vi "ActualizarTabla.vi"(8 "error in (no error)":errorcluster, 11 "Soda Actor in":refnum<class "Soda Actor.lvclass">) -> (0 "error out":errorcluster, 3 "Soda Actor out":refnum<class "Soda Actor.lvclass">)   [LabVIEW 2019, in "Soda Actor.lvlib" / "Soda Actor.lvclass"]
uses:
  Soda Actor.lvclass
  Soda Actor.lvclass/Soda Actor.ctl
  <vilib>/Utility/config.llb/Read Key (Double).vi
  <vilib>/Utility/config.llb/Read Key (String).vi
  <vilib>/Utility/config.llb/NI_LVConfig.lvlib
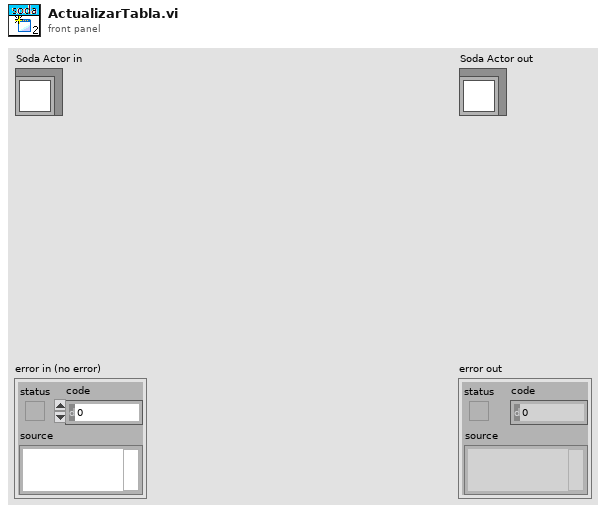
[diagram p1: front panel]
types:
  T1 = typedef "NI_LVConfig.lvlib/Config Data RefNum.ctl" = refnum<k1>
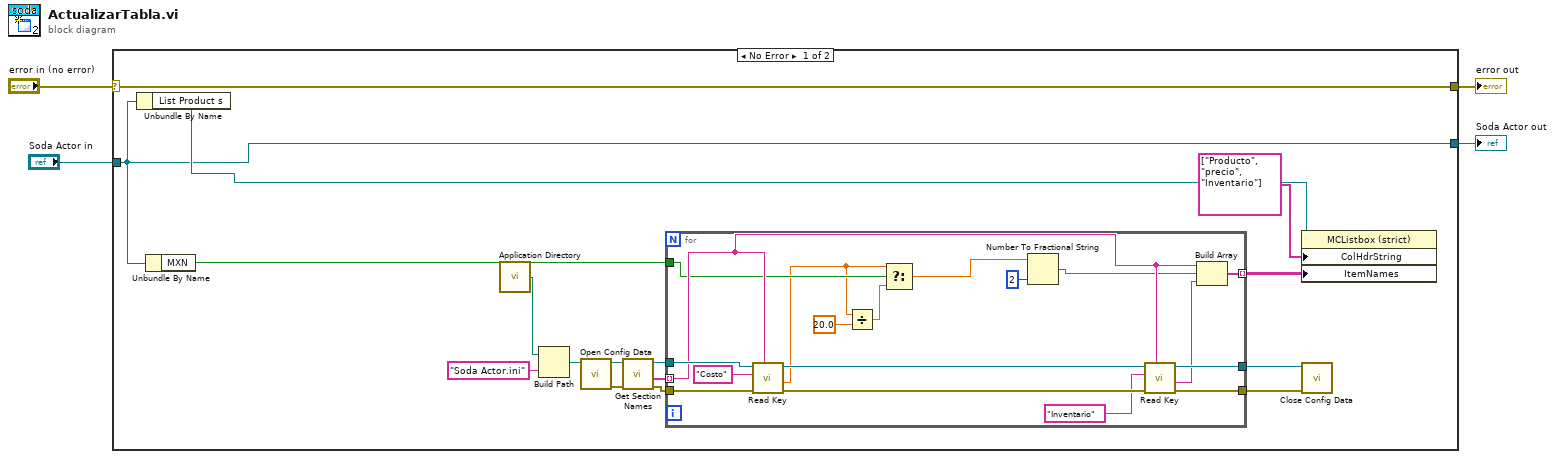
[diagram p0: block diagram]
diagram:
  n1 = case shown="No Error" "error in (no error)" {
    selector: "error in (no error)" -> [w6 w40]
    tunnel: [w6 w40] -> w3
    tunnel: [w15 w39] -> w1
    tunnel: "Soda Actor in" -> [w15 w39]
    frame No Error {
      n2 = Unbundle By Name(w15) -> ("List Product s"=w20:refnum<vi>)
      n3 = Unbundle By Name(w15) -> ("MXN"=w14:bool)
      n4 = call <vilib>:"Application Directory.vi"() -> ("Application Directory"=w19:path)
      n5 = Build Path(base path=w19, name or relative path="Soda Actor.ini") -> (appended path=w18:path)
      n6 = call <vilib>:"Open Config Data.vi"("configuration file path"=w18) -> ("error out"=w11:errorcluster, "refnum"=w12:T1)  [unwired: 8 in, 1 out]
      n7 = call <vilib>:"Get Section Names.vi"("error in (no error)"=w11, "refnum"=w12) -> ("error out"=w9:errorcluster, "section names"=w8:string[], "refnum out"=w10:T1)  [unwired: 7 in]
      n8 = for {
        tunnel: w9 -> [w37]
        tunnel: w10 -> [w38]
        tunnel: [w34] -> w16
        tunnel: [w33] -> w17
        tunnel: w14 -> [w24]
        tunnel: w8 -> [w30] mode=indexing
        tunnel: [w28] -> w7 mode=indexing
        n9 = call-poly <vilib>:"Read Key.vi"("section"=w30, "error in (no error)"=w37, "key"="Costo" ("section"), "refnum"=w38) -> ("error out"=w36:errorcluster, "value"=w23:dbl, "refnum out"=w35:T1)  [unwired: 4 in, 1 out]
        n10 = Divide(x=w23, y=20.0) -> (x/y=w21:dbl)
        n11 = Select(t=w23, s=w24, f=w21) -> (s? t:f=w25:dbl)
        n12 = Number To Fractional String(number=w25, precision (6)=i16 2) -> (F-format string=w27:string)  [unwired: 2 in]
        n13 = call-poly <vilib>:"Read Key.vi"("section"=w30, "error in (no error)"=w36, "key"="Inventario" ("section"), "refnum"=w35) -> ("error out"=w34:errorcluster, "value"=w29:string, "refnum out"=w33:T1)  [unwired: 4 in, 1 out]
        n14 = Build Array(w30, w27, w29) -> (w28:string[])
      }
      n15 = property class="MCListbox (strict)"(reference=w20, "ColHdrString"=string[] ["Producto", "precio", "Inventario"] ("Column Header Strings[]"), "ItemNames"=w7) -> ()  [unwired: 1 in, 2 out]
      n16 = call <vilib>:"Close Config Data.vi"("error in (no error)"=w16, "refnum"=w17) -> ()  [unwired: 8 in, 2 out]
    }
    frame Error {
    }
  }
  "error out" <- w3
  "Soda Actor out" <- w1
